vi "Autonomous Independent.vi"() -> ()   [LabVIEW 2013]
doc: "This VI is called when autonomous begins, and will automatically be terminated when autonomous ends. You can carry out timed or sensor driven robot movement independently without needing to return to the caller."
uses:
  Robot Global Data.vi
  <vilib>/Rock Robotics/WPI/RobotDrive/WPI_RobotDriveGetSetRefNum.vi
  <vilib>/Rock Robotics/WPI/RobotDrive/WPI_RobotDriveArcadeDrive_Standard(NoSaturation).vi
  <vilib>/Rock Robotics/WPI/Solenoid/Deprecated/WPI_SolenoidSetBool.vi
panel:
  out "Current Movement, for debugging":T1 {"Z Joystick Value" scale=-1.0..1.0; "Y Joystick Value" scale=1.0..-1.0; "X Joystick Value" scale=-1.0..1.0}
  in  "Array of robot movements":T2(array[cluster]) {"Z Joystick Value" scale=-1.0..1.0; "Y Joystick Value" scale=1.0..-1.0; "X Joystick Value" scale=-1.0..1.0}
  # "Be sure to right-click and choose Data Operations>>Make Current Value default if you want to save the array values with the VI"
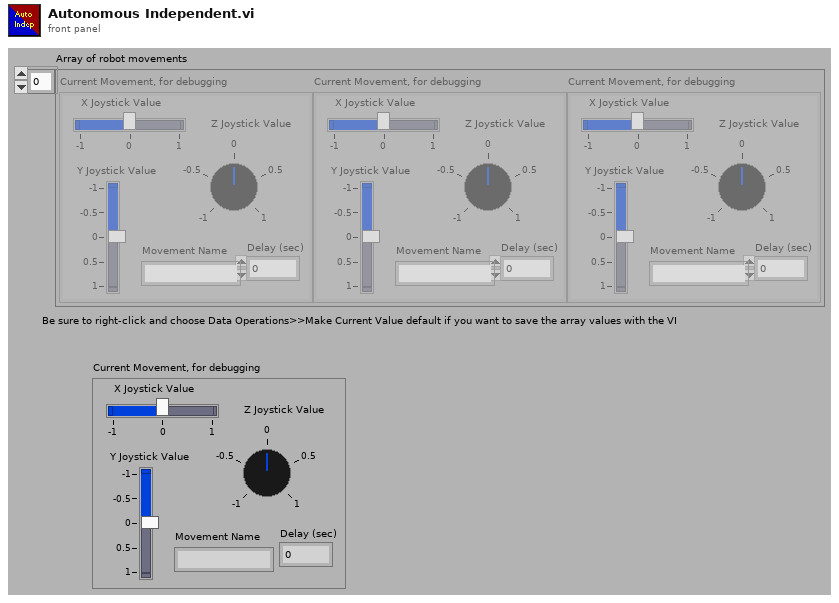
[diagram p1: front panel]
types:
  T1 = cluster{"X Joystick Value":dbl, "Y Joystick Value":dbl, "Z Joystick Value":dbl, "Delay (sec)":dbl, "Movement Name":string}
  T2 = cluster{"X Joystick Value":dbl, "Y Joystick Value":dbl, "Z Joystick Value":dbl, "Delay (sec)":dbl, "Movement Name":string}[]
  T3 = typedef "WPI_RobotDriveDevRef.ctl" = cluster{"DevStatus":errorcluster, "Motors[]":T4[], "Square Inputs":bool, "Max Output":dbl, "Isochronous":bool}
  T4 = typedef "WPI_MotorControlDeviceRef.ctl" = cluster{"DeviceStatus":errorcluster, "Type":enum16{"PWM", "CAN"}, "PWM":cluster{"Digital Module":T5, "PWM Channel":T6, "DeadBand":T7}, "CAN":cluster{"Device Number":u8, "Control Mode":T8, "Semaphore":T9, "Max Vout":dbl}, "Invert":bool, "TransformRef":T10, "InvTransformRef":T10}
  T5 = typedef "FPGA_TypedefDigitalModule.ctl" = enum16{"Digital Module 1", "Digital Module 2"}
  T6 = typedef "FPGA_DIOPWMChannel.ctl" = enum8{"PWM 1", "PWM 2", "PWM 3", "PWM 4", "PWM 5", "PWM 6", "PWM 7", "PWM 8", "PWM 9", "PWM 10", "Invalid"}
  T7 = typedef "WPI_PWMDeadband.ctl" = cluster{"Name":string, "maxPositivePwm":i32, "minPositivePwm":i32, "centerPwm":i32, "maxNegativePwm":i32, "minNegativePwm":i32, "angularRange":u16}
  T8 = typedef "WPI_CANJaguar_ControlMode.ctl" = enum8{"Percent VBus", "Current", "Speed", "Position", "Voltage"}
  T9 = typedef "Semaphore RefNum" = refnum<k1>
  T10 = typedef "WPI_PWMTransform_ConPane.ctl" = refnum<vi>
  T11 = typedef "WPI_SolenoidDevRef.ctl" = cluster{"DevStatus":errorcluster, "Solenoid Module":T12, "Forward Solenoid Channel":T13, "Reverse Solenoid Channel":T13}
  T12 = typedef "FPGA_TypedefSolenoidModule.ctl" = enum16{"Solenoid Module 1", "Solenoid Module 2"}
  T13 = typedef "WPI_SolenoidChannel.ctl" = enum8{"Solenoid 1", "Solenoid 2", "Solenoid 3", "Solenoid 4", "Solenoid 5", "Solenoid 6", "Solenoid 7", "Solenoid 8", "Invalid"}
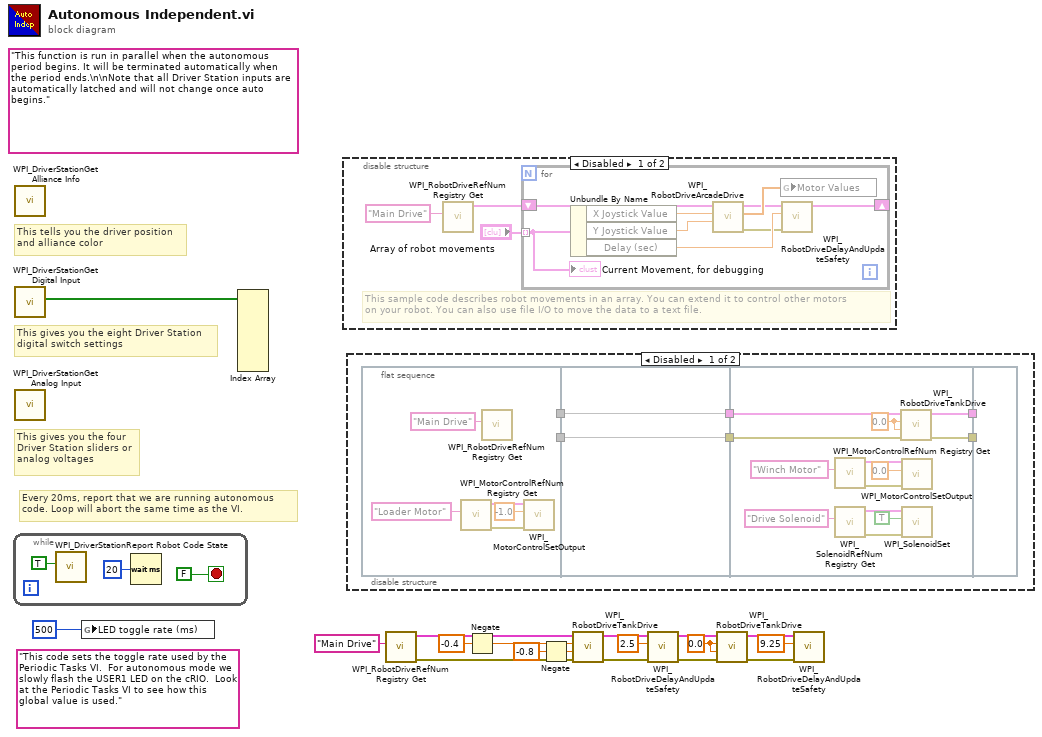
[diagram p0: block diagram]
diagram:
  w10 = 0.0 ("Left axis value")
  (unwired) "This code sets the toggle rate used by the Periodic Tasks VI.  For autonomous mode we slowly flash the USER1 LED on the cRIO.  Look at the Periodic Tasks VI to see how this global value is used."
  (unwired) "This function is run in parallel when the autonomous period begins. It will be terminated automatically when the period ends.\n\nNote that all Driver Station inputs are automatically latched and will not change once auto begins."
  # "Every 20ms, report that we are running autonomous\ncode. Loop will abort the same time as the VI."
  # "This tells you the driver position\nand alliance color"
  # "This gives you the eight Driver Station\ndigital switch settings"
  # "This gives you the four\nDriver Station sliders or\nanalog voltages"
  n1 = while {
    stop <- FALSE stop-if-true
    n2 = call <vilib>:"WPI_DriverStationReport Robot Code State.vi"("Autonomous"=TRUE) -> ()  [unwired: 10 in, 1 out]
    n3 = Wait (ms)(milliseconds to wait=u32 20) -> ()  [unwired: 1 out]
  }
  n4 = call <vilib>:"WPI_DriverStationGet Alliance Info.vi"() -> ()  [unwired: 12 out]
  n5 = call <vilib>:"WPI_DriverStationGet Digital Input.vi"() -> ("Driver Station Digital Input (1-8)"=w18:bool[])  [unwired: 11 out]
  n6 = call <vilib>:"WPI_DriverStationGet Analog Input.vi"() -> ()  [unwired: 12 out]
  n7 = global write "Robot Global Data.vi" "LED toggle rate (ms)"(u32 500 ("LED ms toggle rate")) -> ()
  n8 = Index Array(array=w18) -> ()  [unwired: 8 in, 8 out]
  n9 = disable-structure shown="Disabled" {
    frame Disabled {
      # "This sample code describes robot movements in an array. You can extend it to control other motors\non your robot. You can also use file I/O to move the data to a text file."
      n10 = call <vilib>:"WPI_RobotDriveRefNum Registry Get.vi"("refnum name"="Main Drive") -> ("RobotDriveDevRef"=w23:T3)  [unwired: 1 in, 9 out]
      n11 = for {
        shift-right: [w33] -> _
        shift-left: w23 -> [w30]
        tunnel: "Array of robot movements" -> [w32] mode=indexing
        n12 = Unbundle By Name(w32) -> ("X Joystick Value"=w28:dbl, "Y Joystick Value"=w27:dbl, "Delay (sec)"=w26:dbl)
        n13 = call-poly <vilib>:"WPI_RobotDriveArcadeDrive.vi"("Y axis value"=w27, "X axis value"=w28, "RobotDriveDevRef"=w30) -> ("error out"=w25:errorcluster, "Motor Values"=w31:dbl[], "RobotDriveDevRef"=w29:T3)  [unwired: 6 in]
        n14 = global write "Robot Global Data.vi" "Motor Values"(w31) -> ()
        n15 = call <vilib>:"WPI_RobotDriveDelayAndUpdateSafety.vi"("error in (no error)"=w25, "Delay (s)"=w26, "RobotDriveDevRef"=w29) -> ("RobotDriveDevRef 2"=w33:T3)  [unwired: 7 in, 1 out]
        "Current Movement, for debugging" <- w32
      }
    }
    frame Enabled {
    }
  }
  n16 = disable-structure shown="Disabled" {
    frame Disabled {
      n17 = flat-sequence {
        tunnel: w39 -> [_]
        tunnel: w38 -> [_]
        tunnel: [w46] -> w39
        tunnel: w37 -> [w46]
        tunnel: [w45] -> w38
        tunnel: w36 -> [w45]
        tunnel: [w50] -> w37
        tunnel: [w49] -> w36
        tunnel: [w48] -> w35
        tunnel: [w47] -> w34
        tunnel: w35 -> [_]
        tunnel: w34 -> [_]
        frame #0 {
          n18 = call <vilib>:"WPI_MotorControlRefNum Registry Get.vi"("refnum name"="Loader Motor") -> ("error out"=w43:errorcluster, "MotorControlDevRef"=w41:T4)  [unwired: 9 in]
          n19 = call <vilib>:"WPI_RobotDriveRefNum Registry Get.vi"("refnum name"="Main Drive") -> ()  [unwired: 1 in, 10 out]
          n20 = call <vilib>:"WPI_MotorControlSetOutput.vi"("error in (no error)"=w43, "Output"=-1.0, "MotorControlDevRef"=w41) -> ()  [unwired: 6 in, 3 out]
        }
        frame #1 {
        }
        frame #2 {
          w51 = 0.0 ("Left axis value")
          n21 = call <vilib>:"WPI_MotorControlRefNum Registry Get.vi"("refnum name"="Winch Motor") -> ("error out"=w55:errorcluster, "MotorControlDevRef"=w54:T4)  [unwired: 9 in]
          n22 = call <vilib>:"WPI_SolenoidRefNum Registry Get.vi"("refnum name"="Drive Solenoid") -> ("error out"=w59:errorcluster, "SolenoidDevRef"=w58:T11)  [unwired: 9 in]
          n23 = call <vilib>:"WPI_RobotDriveTankDrive.vi"("error in (no error)"=w49, "Right axis value"=w51, "Left axis value"=w51, "RobotDriveDevRef"=w50) -> ("error out"=w47:errorcluster, "RobotDriveDevRef"=w48:T3)  [unwired: 5 in, 1 out]
          n24 = call <vilib>:"WPI_MotorControlSetOutput.vi"("error in (no error)"=w55, "Output"=0.0, "MotorControlDevRef"=w54) -> ()  [unwired: 6 in, 3 out]
          n25 = call-poly <vilib>:"WPI_SolenoidSet.vi"("error in (no error)"=w59, "Value"=TRUE, "SolenoidDevRef"=w58) -> ()  [unwired: 7 in, 2 out]
        }
        frame #3 {
        }
      }
    }
    frame Enabled {
    }
  }
  n26 = call <vilib>:"WPI_RobotDriveRefNum Registry Get.vi"("refnum name"="Main Drive") -> ("error out"=w14:errorcluster, "RobotDriveDevRef"=w15:T3)  [unwired: 1 in, 8 out]
  n27 = Negate(x=-0.4 ("Left axis value")) -> (-x=w4:dbl)
  n28 = Negate(x=-0.8 ("Right axis value")) -> (-x=w5:dbl)
  n29 = call <vilib>:"WPI_RobotDriveTankDrive.vi"("error in (no error)"=w14, "Right axis value"=w5, "Left axis value"=w4, "RobotDriveDevRef"=w15) -> ("error out"=w11:errorcluster, "RobotDriveDevRef"=w13:T3)  [unwired: 5 in, 1 out]
  n30 = call <vilib>:"WPI_RobotDriveDelayAndUpdateSafety.vi"("error in (no error)"=w11, "Delay (s)"=2.5, "RobotDriveDevRef"=w13) -> ("error out"=w8:errorcluster, "RobotDriveDevRef 2"=w9:T3)  [unwired: 7 in]
  n31 = call <vilib>:"WPI_RobotDriveTankDrive.vi"("error in (no error)"=w8, "Right axis value"=w10, "Left axis value"=w10, "RobotDriveDevRef"=w9) -> ("error out"=w6:errorcluster, "RobotDriveDevRef"=w1:T3)  [unwired: 5 in, 1 out]
  n32 = call <vilib>:"WPI_RobotDriveDelayAndUpdateSafety.vi"("error in (no error)"=w6, "Delay (s)"=9.25, "RobotDriveDevRef"=w1) -> ()  [unwired: 7 in, 2 out]
